vi "Write Sources.vi"(8 "error in (no error)":errorcluster, 10 "Sources":T1[](array[typedef]), 11 "DigitizerBase in":refnum<class "DigitizerBase.lvclass">) -> (0 "error out":errorcluster, 3 "DigitizerBase out":refnum<class "DigitizerBase.lvclass">)   [LabVIEW 2018, in "DigitizerPlugins.lvlib" / "DigitizerBase.lvclass"]
uses:
  DigitizerBase.lvclass
  Typedefs/TrigSource.ctl
  DigitizerBase.lvclass/DigitizerBase.ctl
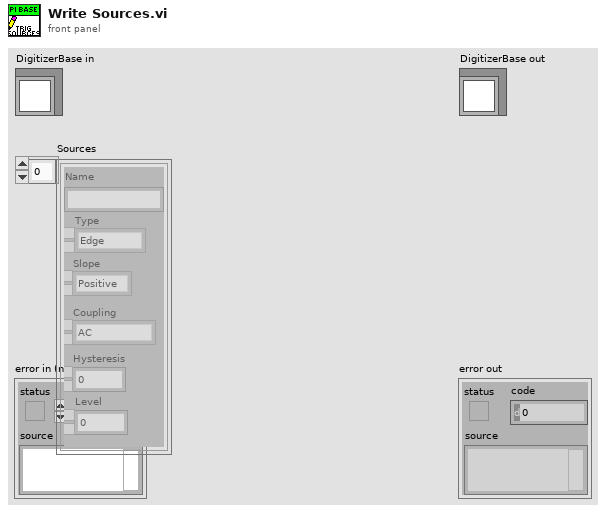
[diagram p1: front panel]
types:
  T1 = typedef "DigitizerPlugins.lvlib/DigitizerBase.lvclass/TrigSource.ctl" = cluster{"Name":string, "Coupling":enum16{"AC", "DC", "HF Reject", "LF Reject", "Noise Reject"}, "Hysteresis":dbl, "Level":dbl, "Slope":enum16{"Positive", "Negative"}, "Type":enum16{"Edge", "Width", "Runt", "Glitch", "TV", "Window"}}
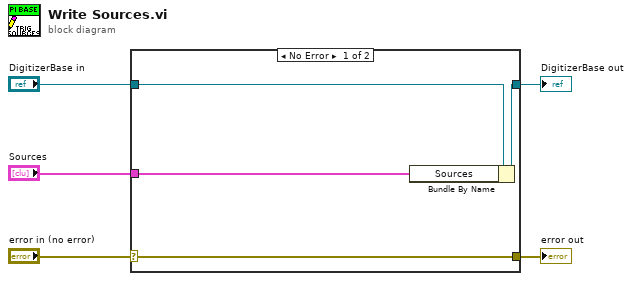
[diagram p0: block diagram]
diagram:
  n1 = case shown="No Error" "error in (no error)" {
    selector: "error in (no error)" -> [w9 w10]
    tunnel: [w9 w10] -> w4
    tunnel: [w7 w11] -> w2
    tunnel: "DigitizerBase in" -> [w8 w11]
    tunnel: "Sources" -> [w6 _]
    frame No Error {
      n2 = Bundle By Name(cluster=w8, "Sources"=w6) -> (w7:refnum<class "DigitizerBase.lvclass">)
    }
    frame Error {
    }
  }
  "error out" <- w4
  "DigitizerBase out" <- w2
